vi "Slave - Interleaved Chs.vi"() -> ()   [LabVIEW 2016]
uses:
  <vilib>/Utility/error.llb/DialogType.ctl
  <vilib>/pximc/Initialize Writer Session (DBL).vi
  <vilib>/pximc/Initialize Reader Session (DBL).vi
  <vilib>/pximc/Connect (DBL).vi
  <vilib>/pximc/Acquire Read Region (DBL).vi
  <vilib>/pximc/Acquire Write Region (DBL).vi
  <vilib>/pximc/nipximc.lvlib
panel:
  out "Stopped?":bool=TRUE
  in  "Stop Button":bool
  in  "#Reading Channels":i32=8
  in  "#Writing Channels Slave 2":i32=4
  out "Waveform Chart 2":T1(graph)={"[0]"=0.35836794954530016, "[1]"=-0.8660254037842426, "[2]"=0.8910065241883677, "[3]"=0.0, "[4]"=0.9945218953682733, "[5]"=0.25881904510249687, "[6]"=0.544639035015028, "[7]"=0.0, "[8]"=0.0}
  in  "#Reading Channels":i32=8
  in  "#Writing Channels Slave 1":i32=4
  out "Waveform Chart 1":T1(graph)={"[0]"=0.8090169943749952, "[1]"=-0.17364817766690352, "[2]"=0.0, "[3]"=-0.866025403784546, "[4]"=0.6156614753256503, "[5]"=0.0, "[6]"=0.34202014332579517, "[7]"=-0.7660444431189357, "[8]"=0.0}
  in  "Node 1 Reader Connection ID":u16=4
  in  "Reader Interface Node 2":tag="PXIMC2" caption="interface"
  in  "Node 2 Writer Connection ID":u16=3
  in  "Writer Interface Node 2":tag="PXIMC2" caption="interface"
  in  "Node 1 Writer Connection ID":u16=1
  in  "Node 1 Writer Interface":tag="PXIMC2" caption="interface"
  in  "Node 1 Reader Interface":tag="PXIMC2" caption="interface"
  in  "Buffer Size":u64=250000 caption="buffer size"
  in  "Connection Timeout (s)":dbl=60.0 caption="timeout in seconds (-1)"
  in  "Node 1 Reader Connection ID":u16=2
  # "Node 1"
  # "Node 2"
  # "Node 2 => Node 1"
  # "Node 1 => Node 2"
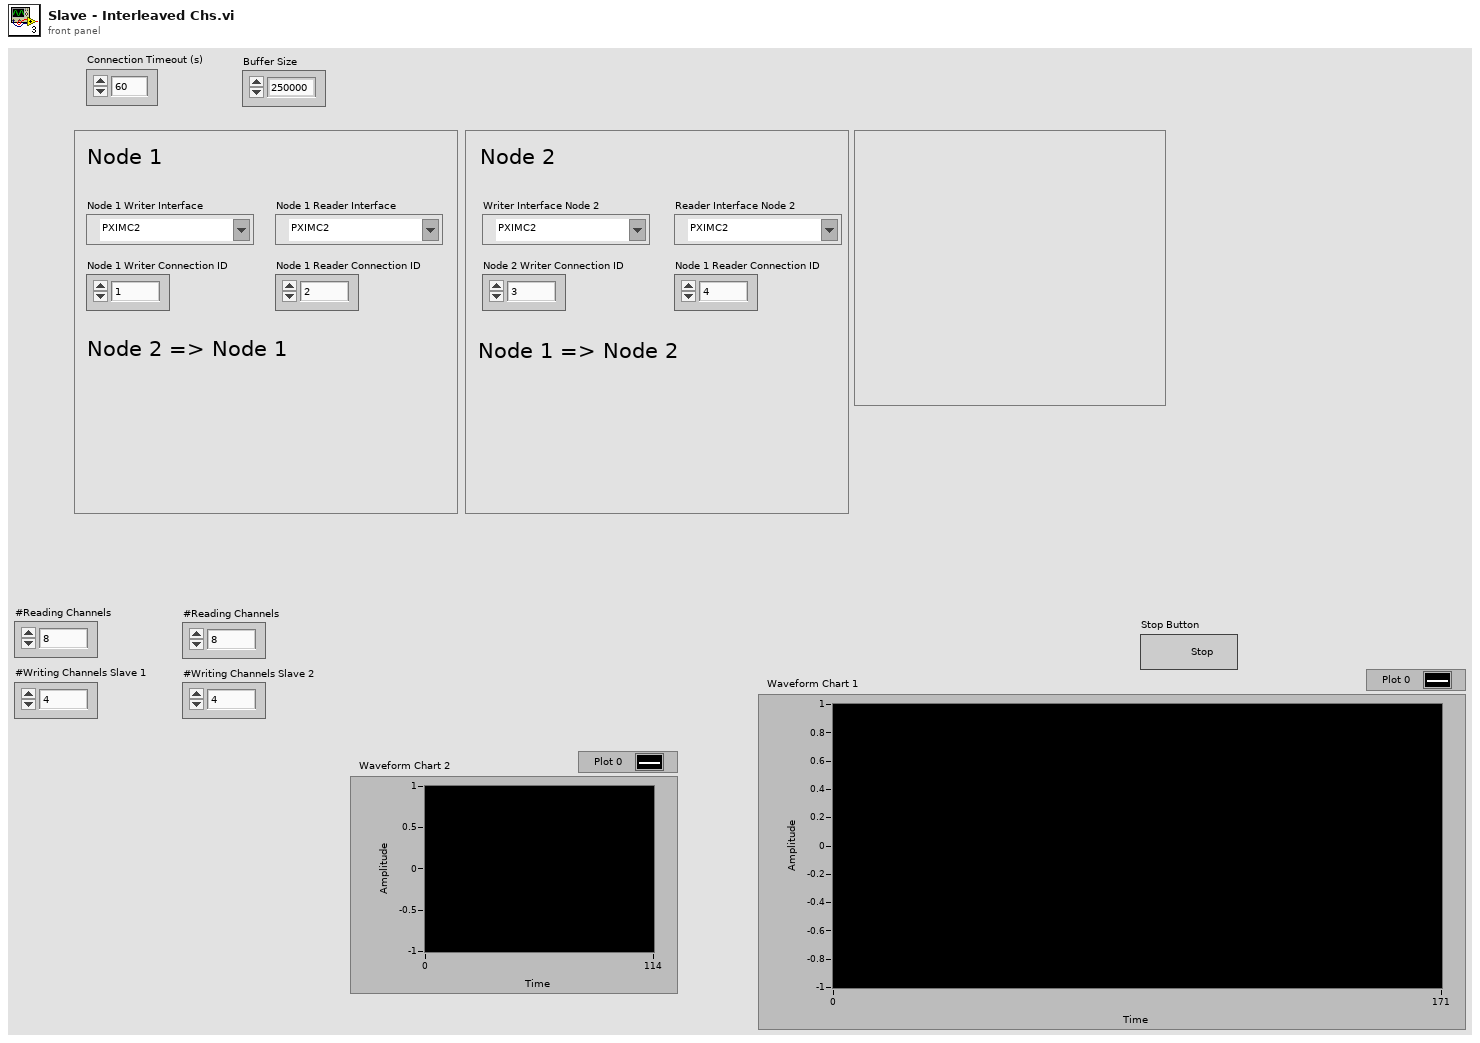
[diagram p1: front panel]
types:
  T1 = cluster{"[0]":dbl, "[1]":dbl, "[2]":dbl, "[3]":dbl, "[4]":dbl, "[5]":dbl, "[6]":dbl, "[7]":dbl, "[8]":dbl}
  T2 = typedef "DialogType.ctl" = u16
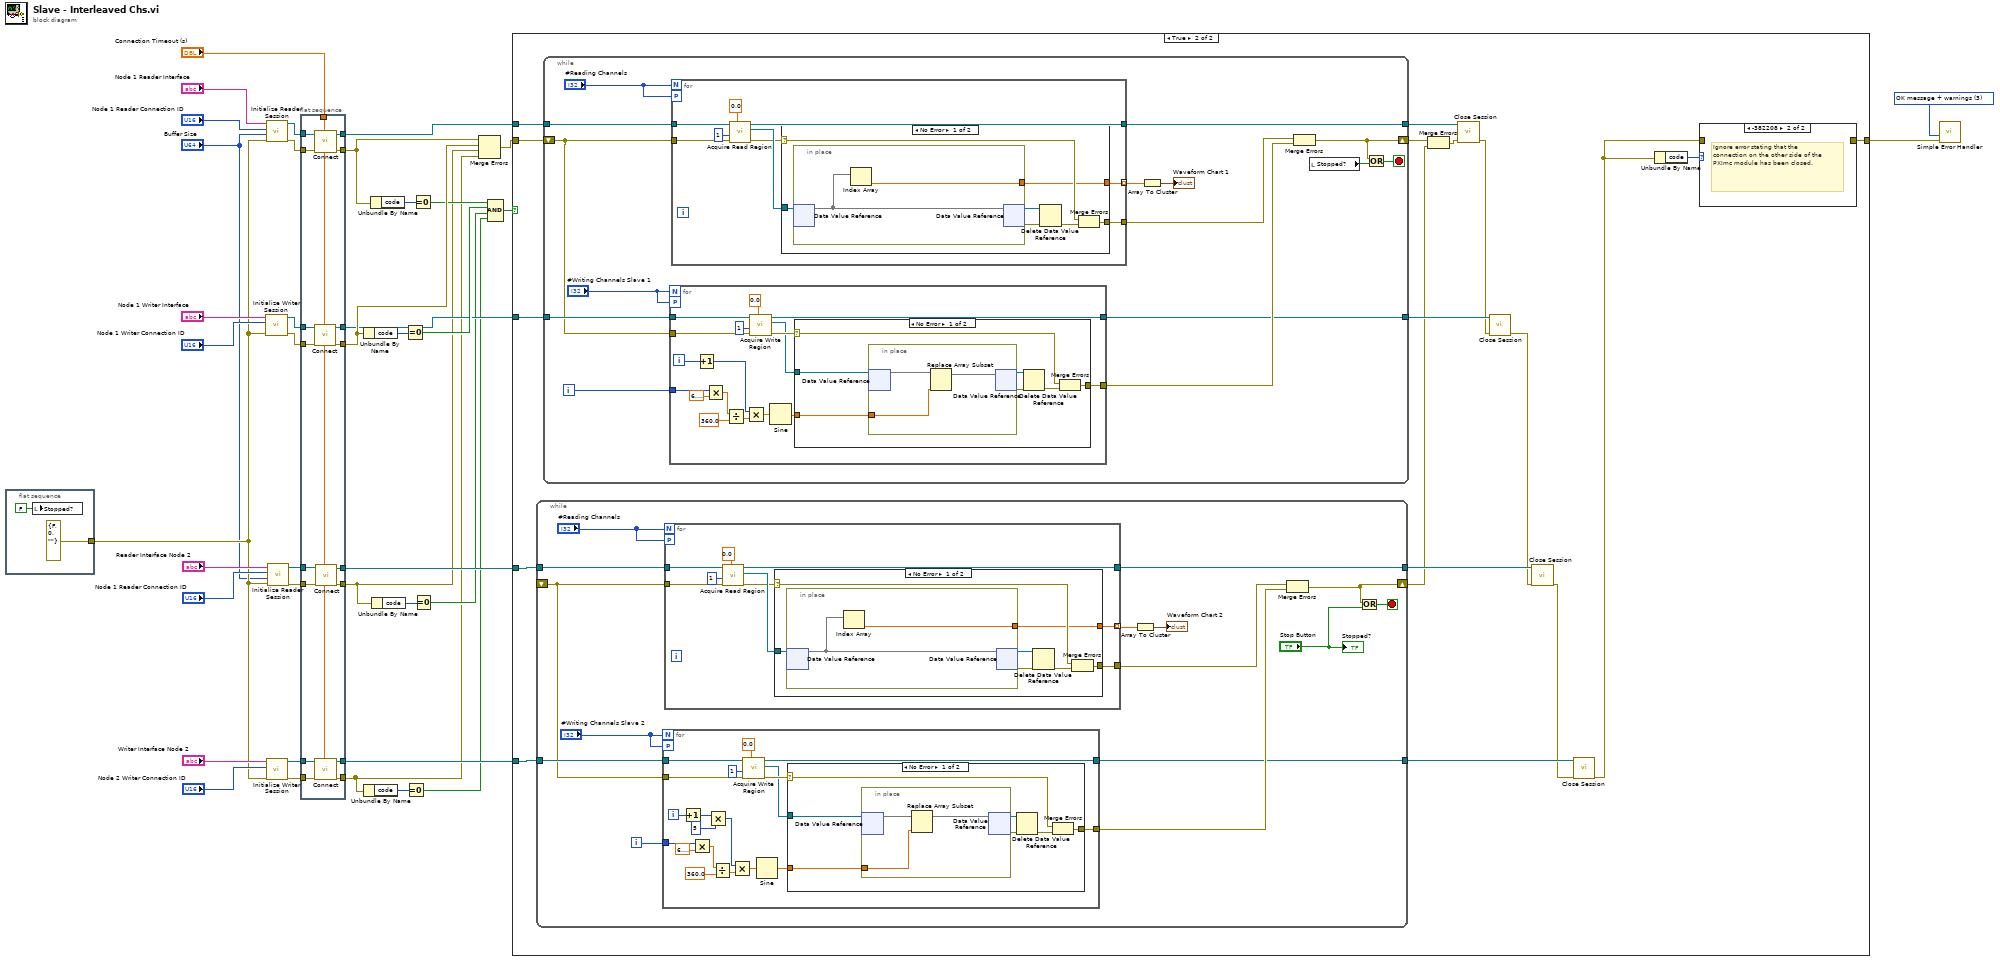
[diagram p0: block diagram]
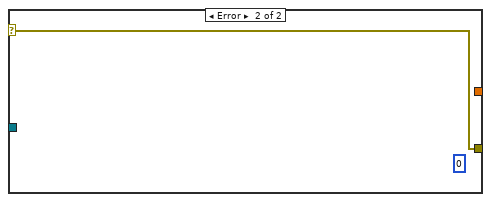
[diagram p3: hidden frame]
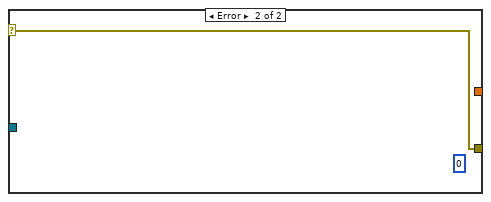
[diagram p5: hidden frame]
diagram:
  w33 = T2 3 items=["no dialog", "OK message", "continue or stop message", "OK message + warnings", "continue/stop + warnings"] ("type of dialog (OK msg:1)")
  n1 = flat-sequence {
    tunnel: [errorcluster {"status"=FALSE, "code"=0, "source"=""} ("error constant")] -> w10
    frame #0 {
      n2 = local write "Stopped?"(FALSE ("Stopped?")) -> ()
    }
  }
  n3 = call-poly <vilib>:"Initialize Writer Session.vi"("error in (no error)"=w10, "connection id (1)"="Node 1 Writer Connection ID", "interface"="Node 1 Writer Interface") -> ("error out"=w31:errorcluster, "session out"=w30:refnum<k21>)  [unwired: 7 in]
  n4 = call-poly <vilib>:"Initialize Reader Session.vi"("error in (no error)"=w10, "buffer size"="Buffer Size", "writer's connection id (1)"="Node 1 Reader Connection ID", "interface"="Node 1 Reader Interface") -> ("error out"=w37:errorcluster, "session out"=w38:refnum<k21>)  [unwired: 6 in]
  n5 = call-poly <vilib>:"Initialize Writer Session.vi"("error in (no error)"=w10, "connection id (1)"="Node 2 Writer Connection ID", "interface"="Writer Interface Node 2") -> ("error out"=w17:errorcluster, "session out"=w18:refnum<k21>)  [unwired: 7 in]
  n6 = call-poly <vilib>:"Initialize Reader Session.vi"("error in (no error)"=w10, "buffer size"="Buffer Size", "writer's connection id (1)"="Node 1 Reader Connection ID", "interface"="Reader Interface Node 2") -> ("error out"=w13:errorcluster, "session out"=w12:refnum<k21>)  [unwired: 6 in]
  n7 = flat-sequence {
    tunnel: w38 -> [w58]
    tunnel: w37 -> [w57]
    tunnel: [w56] -> w36
    tunnel: w31 -> [w55]
    tunnel: w30 -> [w54]
    tunnel: [w53] -> w24
    tunnel: [w52] -> w23
    tunnel: "Connection Timeout (s)" -> [w42]
    tunnel: [w51] -> w21
    tunnel: [w50] -> w5
    tunnel: [w49] -> w1
    tunnel: [w48] -> w2
    tunnel: w18 -> [w47]
    tunnel: w17 -> [w46]
    tunnel: [w45] -> w6
    tunnel: w13 -> [w44]
    tunnel: w12 -> [w43]
    frame #0 {
      n8 = call-poly <vilib>:"Connect.vi"("timeout in seconds (-1)"=w42, "error in (no error)"=w55, "session in"=w54) -> ("error out"=w52:errorcluster, "session out"=w51:refnum<k21>)  [unwired: 7 in]
      n9 = call-poly <vilib>:"Connect.vi"("timeout in seconds (-1)"=w42, "error in (no error)"=w57, "session in"=w58) -> ("error out"=w53:errorcluster, "session out"=w56:refnum<k21>)  [unwired: 7 in]
      n10 = call-poly <vilib>:"Connect.vi"("timeout in seconds (-1)"=w42, "error in (no error)"=w46, "session in"=w47) -> ("error out"=w49:errorcluster, "session out"=w50:refnum<k21>)  [unwired: 7 in]
      n11 = call-poly <vilib>:"Connect.vi"("timeout in seconds (-1)"=w42, "error in (no error)"=w44, "session in"=w43) -> ("error out"=w48:errorcluster, "session out"=w45:refnum<k21>)  [unwired: 7 in]
    }
  }
  n12 = Unbundle By Name(w23) -> ("code"=w28:i32)
  n13 = Unbundle By Name(w1) -> ("code"=w20:i32)
  n14 = Unbundle By Name(w24) -> ("code"=w34:i32)
  n15 = Unbundle By Name(w2) -> ("code"=w15:i32)
  n16 = Equal To 0?(x=w28) -> (x = 0?=w26:bool)
  n17 = Equal To 0?(x=w20) -> (x = 0?=w3:bool)
  n18 = Equal To 0?(x=w34) -> (x = 0?=w8:bool)
  n19 = Equal To 0?(x=w15) -> (x = 0?=w4:bool)
  n20 = Merge Errors(w24, w23, w2, w1) -> (w25:errorcluster)
  n21 = Compound Arithmetic op=AND(w8, w26, w4, w3) -> (w27:bool)
  n22 = case shown="True" w27 {
    tunnel: w25 -> [w59 w60]
    tunnel: w36 -> [_ w73]
    tunnel: [w59 w77] -> w7
    tunnel: w21 -> [_ w72]
    tunnel: w6 -> [_ w75]
    tunnel: w5 -> [_ w74]
    frame False {
      # "The connection was not successful for some reason."
    }
    frame True {
      n23 = while {
        tunnel: w75 -> [w85]
        tunnel: [w84] -> w69
        shift-right: [w91] -> w62
        shift-left: _ -> [w79]
        tunnel: w74 -> [w90]
        tunnel: [w81] -> w67
        i -> [w78]
        stop <- w92 stop-if-true
        n24 = for {
          N: "#Writing Channels Slave 2" -> [_]
          tunnel: w90 -> [w130]
          tunnel: [w129] -> w81
          tunnel: [w127] -> w82
          workers-P: "#Writing Channels Slave 2" -> [_]
          tunnel: w79 -> [w124]
          tunnel: w78 -> [w116]
          i -> [w117]
          n25 = Increment(x=w117) -> (x+1=w114:i32)
          n26 = Multiply(x=w116, y=6.283185307179586) -> (x*y=w121:dbl)
          n27 = Multiply(x=w114, y=5) -> (x*y=w112:i32)
          n28 = Divide(x=w121, y=360.0) -> (x/y=w119:dbl)
          n29 = Multiply(x=w112, y=w119) -> (x*y=w118:dbl)
          n30 = call-poly <vilib>:"Acquire Write Region.vi"("timeout in seconds (5)"=0.0, "error in (no error)"=w124, "number of elements"=1, "session in"=w130) -> ("error out"=w128:errorcluster, "write region reference"=w126:refnum<data-value>, "session out"=w129:refnum<k21>)  [unwired: 4 in, 1 out]
          n31 = Sine(x=w118) -> (sin(x)=w115:dbl)
          n32 = case shown="No Error" w128 {
            selector: w128 -> [w133 w141]
            tunnel: w126 -> [w137 _]
            tunnel: [w134 w141] -> w127
            tunnel: w115 -> [w131 _]
            frame No Error {
              n33 = in-place {
                in-place-border: w131 -> [w139]
                n34 = in-place-dvr #1(w137) -> (w140:dbl[])  [unwired: 1 out]
                n35 = Replace Array Subset(array=w140, new element=w139) -> (w138:dbl[])  [unwired: 1 in]
                n36 = in-place-dvr #1(w138) -> (w136:refnum<data-value>, w135:errorcluster)
              }
              n37 = Delete Data Value Reference(data value reference=w136, error in=w135) -> (error out=w132:errorcluster)  [unwired: 1 out]
              n38 = Merge Errors(w133, w132) -> (w134:errorcluster)
            }
            frame Error {
            }
          }
        }
        n39 = for {
          N: "#Reading Channels" -> [_]
          tunnel: [w100] -> w84
          tunnel: w85 -> [w99]
          tunnel: w79 -> [w98]
          tunnel: [w97] -> w83
          workers-P: "#Reading Channels" -> [_]
          tunnel: [w94] -> w87 mode=indexing
          n40 = call-poly <vilib>:"Acquire Read Region.vi"("timeout in seconds (5)"=0.0, "error in (no error)"=w98, "number of elements"=1, "session in"=w99) -> ("error out"=w96:errorcluster, "read region reference"=w101:refnum<data-value>, "session out"=w100:refnum<k21>)  [unwired: 4 in, 1 out]
          n41 = case shown="No Error" w96 {
            selector: w96 -> [w104 w111]
            tunnel: w101 -> [w108 _]
            tunnel: [w103 w111] -> w97
            tunnel: [w102 _] -> w94
            frame No Error {
              n42 = in-place {
                in-place-border: [w109] -> w102
                n43 = in-place-dvr #2(w108) -> (w110:dbl[])  [unwired: 1 out]
                n44 = Index Array(array=w110) -> (element=w109:dbl)  [unwired: 1 in]
                n45 = in-place-dvr #2(w110) -> (w107:refnum<data-value>, w106:errorcluster)
              }
              n46 = Delete Data Value Reference(data value reference=w107, error in=w106) -> (error out=w105:errorcluster)  [unwired: 1 out]
              n47 = Merge Errors(w104, w105) -> (w103:errorcluster)
            }
            frame Error {
              (unwired) u64 0
            }
          }
        }
        n48 = Array To Cluster(array=w87) -> (cluster=→"Waveform Chart 2":T1)
        n49 = Merge Errors(w83, w82) -> (w91:errorcluster)
        n50 = Or(x=w91, y="Stop Button") -> (x .or. y?=w92:bool)
        "Stopped?" <- "Stop Button"
      }
      n51 = while {
        tunnel: [w149] -> w64
        shift-right: [w155] -> w63
        shift-left: w60 -> [w143]
        tunnel: w73 -> [w146]
        tunnel: w72 -> [w145]
        tunnel: [w144] -> w71
        i -> [w142]
        stop <- w156 stop-if-true
        n52 = for {
          N: "#Writing Channels Slave 1" -> [_]
          tunnel: w145 -> [w192]
          tunnel: [w191] -> w144
          tunnel: [w189] -> w147
          workers-P: "#Writing Channels Slave 1" -> [_]
          tunnel: w143 -> [w186]
          tunnel: w142 -> [w180]
          i -> [w178]
          n53 = Increment(x=w178) -> (x+1=w177:i32)
          n54 = Multiply(x=w180, y=6.283185307179586) -> (x*y=w183:dbl)
          n55 = Divide(x=w183, y=360.0) -> (x/y=w179:dbl)
          n56 = Multiply(x=w177, y=w179) -> (x*y=w176:dbl)
          n57 = call-poly <vilib>:"Acquire Write Region.vi"("timeout in seconds (5)"=0.0, "error in (no error)"=w186, "number of elements"=1, "session in"=w192) -> ("error out"=w190:errorcluster, "write region reference"=w188:refnum<data-value>, "session out"=w191:refnum<k21>)  [unwired: 4 in, 1 out]
          n58 = Sine(x=w176) -> (sin(x)=w181:dbl)
          n59 = case shown="No Error" w190 {
            selector: w190 -> [w195 w203]
            tunnel: w188 -> [w199 _]
            tunnel: [w196 w203] -> w189
            tunnel: w181 -> [w193 _]
            frame No Error {
              n60 = in-place {
                in-place-border: w193 -> [w200]
                n61 = in-place-dvr #3(w199) -> (w202:dbl[])  [unwired: 1 out]
                n62 = Replace Array Subset(array=w202, new element=w200) -> (w201:dbl[])  [unwired: 1 in]
                n63 = in-place-dvr #3(w201) -> (w198:refnum<data-value>, w197:errorcluster)
              }
              n64 = Delete Data Value Reference(data value reference=w198, error in=w197) -> (error out=w194:errorcluster)  [unwired: 1 out]
              n65 = Merge Errors(w195, w194) -> (w196:errorcluster)
            }
            frame Error {
            }
          }
        }
        n66 = for {
          N: "#Reading Channels" -> [_]
          tunnel: [w164] -> w149
          tunnel: w146 -> [w163]
          tunnel: w143 -> [w162]
          tunnel: [w161] -> w148
          workers-P: "#Reading Channels" -> [_]
          tunnel: [w158] -> w151 mode=indexing
          n67 = call-poly <vilib>:"Acquire Read Region.vi"("timeout in seconds (5)"=0.0, "error in (no error)"=w162, "number of elements"=1, "session in"=w163) -> ("error out"=w160:errorcluster, "read region reference"=w165:refnum<data-value>, "session out"=w164:refnum<k21>)  [unwired: 4 in, 1 out]
          n68 = case shown="No Error" w160 {
            selector: w160 -> [w168 w175]
            tunnel: w165 -> [w172 _]
            tunnel: [w167 w175] -> w161
            tunnel: [w166 _] -> w158
            frame No Error {
              n69 = in-place {
                in-place-border: [w173] -> w166
                n70 = in-place-dvr #4(w172) -> (w174:dbl[])  [unwired: 1 out]
                n71 = Index Array(array=w174) -> (element=w173:dbl)  [unwired: 1 in]
                n72 = in-place-dvr #4(w174) -> (w171:refnum<data-value>, w170:errorcluster)
              }
              n73 = Delete Data Value Reference(data value reference=w171, error in=w170) -> (error out=w169:errorcluster)  [unwired: 1 out]
              n74 = Merge Errors(w168, w169) -> (w167:errorcluster)
            }
            frame Error {
              (unwired) u64 0
            }
          }
        }
        n75 = Array To Cluster(array=w151) -> (cluster=→"Waveform Chart 1":T1)
        n76 = Merge Errors(w148, w147) -> (w155:errorcluster)
        n77 = local read "Stopped?"() -> (w154:bool)
        n78 = Or(x=w155, y=w154) -> (x .or. y?=w156:bool)
      }
      n79 = Merge Errors(w63, w62) -> (w61:errorcluster)
      n80 = call <vilib>:"Close Session.vi"("error in (no error)"=w61, "session in"=w64) -> ("error out"=w70:errorcluster)  [unwired: 9 in]
      n81 = call <vilib>:"Close Session.vi"("error in (no error)"=w70, "session in"=w71) -> ("error out"=w68:errorcluster)  [unwired: 9 in]
      n82 = call <vilib>:"Close Session.vi"("error in (no error)"=w68, "session in"=w69) -> ("error out"=w66:errorcluster)  [unwired: 9 in]
      n83 = call <vilib>:"Close Session.vi"("error in (no error)"=w66, "session in"=w67) -> ("error out"=w65:errorcluster)  [unwired: 9 in]
      n84 = Unbundle By Name(w65) -> ("code"=w76:i32)
      n85 = case shown="-382208" w76 {
        tunnel: w65 -> [w204 _]
        tunnel: [w204 _] -> w77
        frame 0, Default {
        }
        frame -382208 {
          # "Ignore error stating that the connection on the other side of the PXImc module has been closed."
        }
      }
    }
  }
  n86 = call <vilib>:"Simple Error Handler.vi"("type of dialog (OK msg:1)"=w33, "error in (no error)"=w7) -> ()  [unwired: 3 in, 5 out]
